vi "Pockels Cal-Cancel handler.vi"() -> (3 "Stop?":bool)   [LabVIEW 2013]
uses:
  Globals/gl_Calibration globals.vi
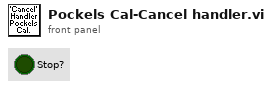
[diagram p1: front panel]
types:
  T1 = typedef "Pockels cal process refs.ctl" = cluster{"This VI":refnum<vi>, "Abort (ind)":refnum<vi>, "Next (ind)":refnum<vi>, "Cancel":refnum<vi>, "Next":refnum<vi>, "Message":refnum<vi>, "Measured Power ctrl":refnum<vi>, "Measured Power ind":refnum<vi>, "Pockels cal progress bar":refnum<vi>, "Abort this objective":refnum<vi>}
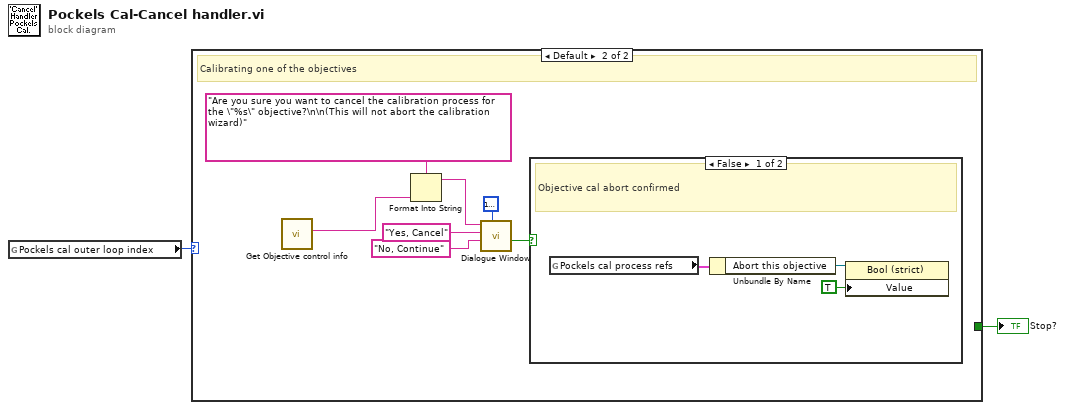
[diagram p0: block diagram]
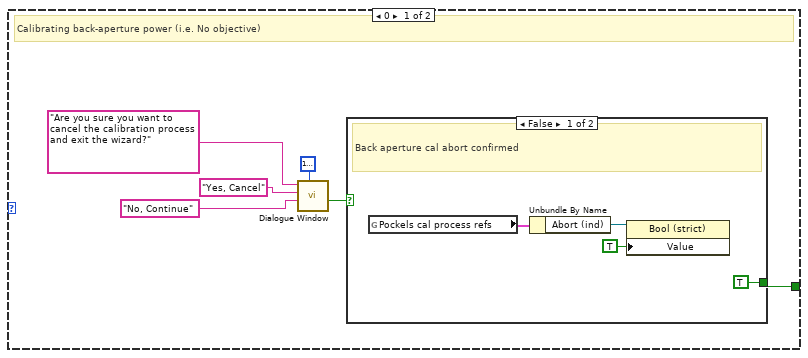
[diagram p2: hidden frame]
diagram:
  n1 = global read "gl_Calibration globals.vi" "Pockels cal outer loop index"() -> (w1:i32)
  n2 = case shown="Default" w1 {
    tunnel: [w8 _] -> w2
    frame 0 {
      # "Calibrating back-aperture power (i.e. No objective)"
      n3 = call "Dialogue Window.vi"("Colour"=u32 16777225, "Caption-Left button (Cancel)"="No, Continue", "Caption-Right button (OK)"="Yes, Cancel", "Message string"="Are you sure you want to cancel the calibration process and exit the wizard?") -> ("Cancelled (Left button pressed)"=w7:bool)  [unwired: 5 in, 2 out]
      n4 = case shown="False" w7 {
        tunnel: [TRUE ("Stop?") _] -> w8
        frame False {
          # "Back aperture cal abort confirmed"
          n5 = global read "gl_Calibration globals.vi" "Pockels cal process refs"() -> (w10:T1)
          n6 = Unbundle By Name(w10) -> ("Abort (ind)"=w9:refnum<vi>)
          n7 = property class="Bool (strict)"(reference=w9, "Value"=TRUE) -> ()  [unwired: 1 in, 2 out]
        }
        frame True {
          # "Abort was cancelled..\nSo continue"
        }
      }
    }
    frame Default {
      # "Calibrating one of the objectives"
      n8 = call "Get Objective control info.vi"() -> ("Value"=w13:string)  [unwired: 7 in, 4 out]
      n9 = Format Into String(format string="Are you sure you want to cancel the calibration process for the \"%s\" objective?\n\n(This will not abort the calibration wizard)" ("Message string"), w13) -> (resulting string=w14:string)  [unwired: 2 in, 1 out]
      n10 = call "Dialogue Window.vi"("Colour"=u32 16777225, "Caption-Left button (Cancel)"="No, Continue", "Caption-Right button (OK)"="Yes, Cancel", "Message string"=w14) -> ("Cancelled (Left button pressed)"=w19:bool)  [unwired: 5 in, 2 out]
      n11 = case shown="False" w19 {
        frame False {
          # "Objective cal abort confirmed"
          n12 = global read "gl_Calibration globals.vi" "Pockels cal process refs"() -> (w21:T1)
          n13 = Unbundle By Name(w21) -> ("Abort this objective"=w20:refnum<vi>)
          n14 = property class="Bool (strict)"(reference=w20, "Value"=TRUE) -> ()  [unwired: 1 in, 2 out]
        }
        frame True {
          # "Abort was cancelled..\nSo continue"
        }
      }
    }
  }
  "Stop?" <- w2
